vi "get_destination.vi"(0 "HGF_ThreadTask":refnum<class "HGF_ThreadTask.lvclass">, 5 "error in (no error)":errorcluster) -> (14 "dup HGF_ThreadTask":refnum<class "HGF_ThreadTask.lvclass">, 16 "destination":refnum<class "HGF_Event.lvclass">, 19 "error out":errorcluster)   [LabVIEW 2014, in "HGF_BaseClasses.lvlib" / "HGF_ThreadTask.lvclass"]
doc: "Read destinationEvent."
uses:
  HGF_ThreadTask.lvclass
  HGF_Event/HGF_Event.lvclass
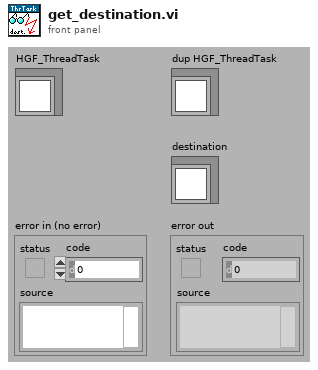
[diagram p1: front panel]
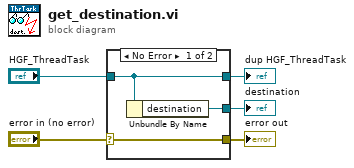
[diagram p0: block diagram]
diagram:
  n1 = case shown="No Error" "error in (no error)" {
    selector: "error in (no error)" -> [w8 w9]
    tunnel: [w8 w9] -> w4
    tunnel: [w7 w10] -> w2
    tunnel: "HGF_ThreadTask" -> [w7 w10]
    tunnel: [w6 _] -> w1
    frame No Error {
      n2 = Unbundle By Name(w7) -> ("destination"=w6:refnum<class "HGF_Event.lvclass">)
    }
    frame Error {
    }
  }
  "error out" <- w4
  "dup HGF_ThreadTask" <- w2
  "destination" <- w1
